vi "Internal Operation.vi"(7 "Archt Map":variant, 9 "Message":T2, 10 "ThreadData":T1={"AUTO_ERROR_HANDLE"={"ENABLE"=FALSE, "ANCHOR"="cleanup"}}, 11 "Numeric in":i32) -> (0 "error out":errorcluster, 2 "ThreadData (dup)":T1={"AUTO_ERROR_HANDLE"={"ENABLE"=FALSE, "ANCHOR"="cleanup"}}, 3 "Numeric out":i32)   [LabVIEW 2020, in "CSMScript-Engine(Lite).lvlib"]
uses:
  CSMScript-Engine(Lite).lvlib
  <userlib>/_NEVSTOP/Communicable State Machine(CSM)/addons/API-String-Arugments-Support/API String Arguments Support.lvlib
  <userlib>/_NEVSTOP/Communicable State Machine(CSM)/_Shared/CSM Shared.lvlib
  Typedef/Def-Thread Data.ctl
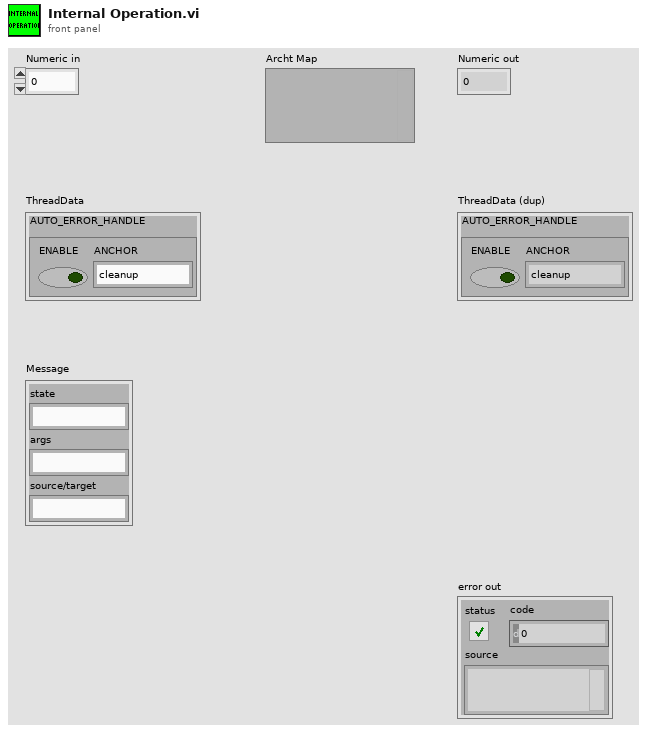
[diagram p1: front panel]
types:
  T1 = typedef "CSMScript-Engine(Lite).lvlib/Def-Thread Data.ctl" = cluster{"AUTO_ERROR_HANDLE":cluster{"ENABLE":bool, "ANCHOR":string}}
  T2 = cluster{"state":string, "args":string, "source/target":string}
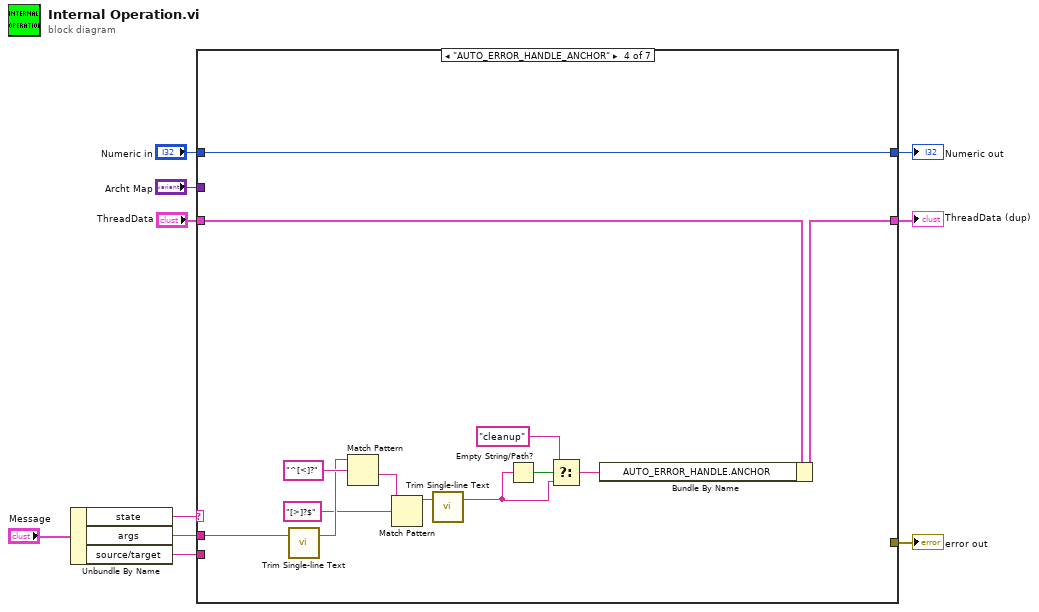
[diagram p0: block diagram]
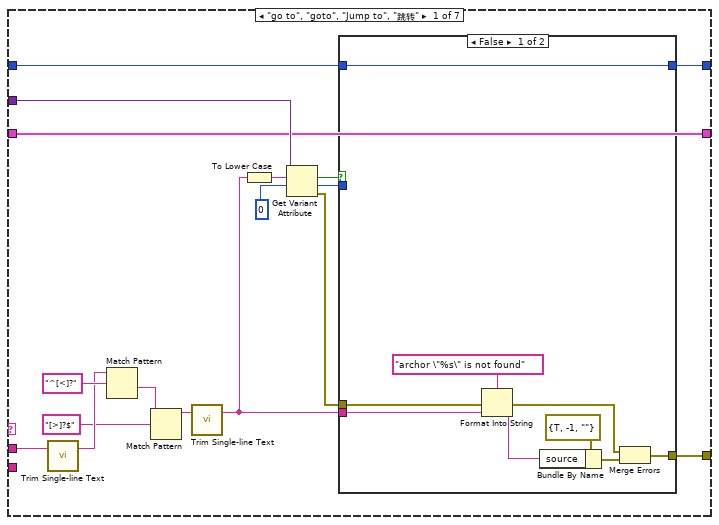
[diagram p2: hidden frame]
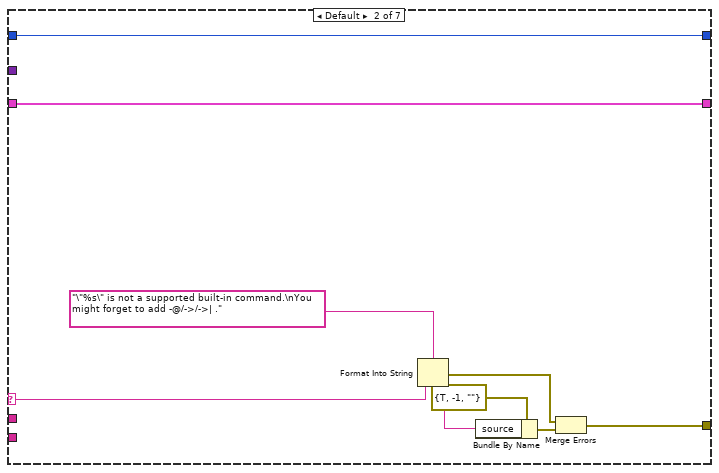
[diagram p4: hidden frame]
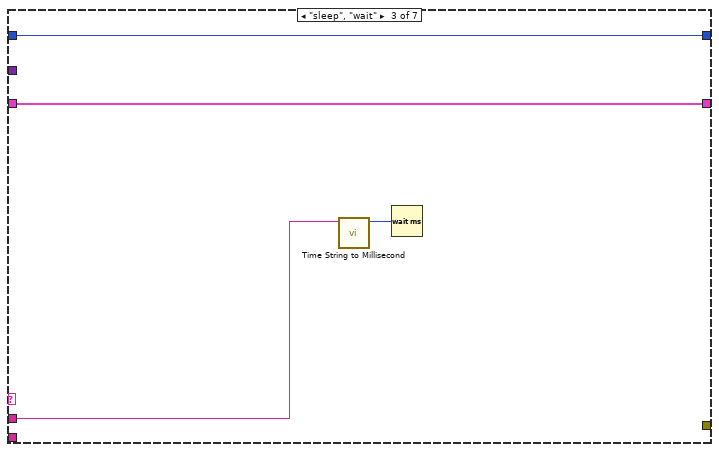
[diagram p5: hidden frame]
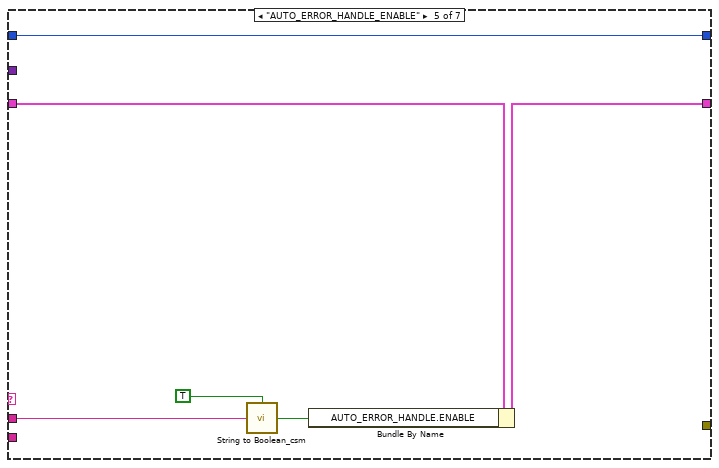
[diagram p6: hidden frame]
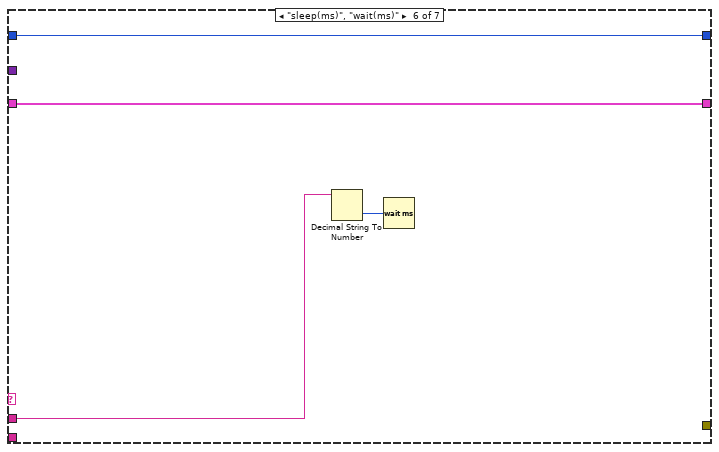
[diagram p7: hidden frame]
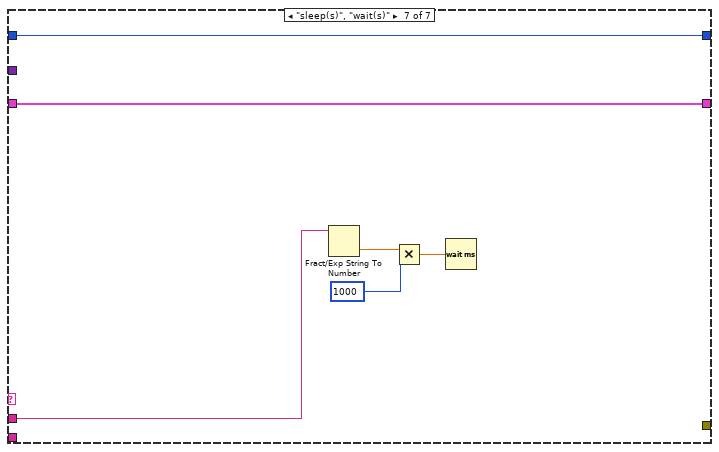
[diagram p8: hidden frame]
diagram:
  n1 = Unbundle By Name("Message") -> ("state"=w5:string, "args"=w4:string, "source/target"=w3:string)
  n2 = case shown="\"AUTO_ERROR_HANDLE_ANCHOR\"" w5 {
    selector: w5 -> [_ w39 _ _ _ _ _]
    tunnel: w4 -> [w17 _ w49 w52 w66 w72 w78]
    tunnel: [w24 w46 w50 w63 w69 w73 w79] -> w7
    tunnel: "Numeric in" -> [w23 w46 w50 w63 w69 w73 w79]
    tunnel: "Archt Map" -> [w27 _ _ _ _ _ _]
    tunnel: [w21 w40 _ _ _ _ _] -> w10
    tunnel: w3 -> [_ _ _ _ _ _ _]
    tunnel: "ThreadData" -> [w18 w38 w47 w62 w68 w70 w74]
    tunnel: [w18 w38 w47 w61 w67 w70 w74] -> w1
    frame "go to", "goto", "Jump to", "跳转" {
      n3 = call <userlib>:"Trim Single-line Text.vi"("single-line text"=w17) -> ("trimed text"=w15:string)  [unwired: 2 in]
      n4 = Match Pattern(string=w15, regular expression="^[<]?") -> (after substring=w13:string)  [unwired: 1 in, 3 out]
      n5 = Match Pattern(string=w13, regular expression="[>]?$") -> (before substring=w12:string)  [unwired: 1 in, 3 out]
      n6 = call <userlib>:"Trim Single-line Text.vi"("single-line text"=w12) -> ("trimed text"=w11:string)  [unwired: 2 in]
      n7 = To Lower Case(string=w11) -> (all lower case string=w19:string)
      n8 = Get Variant Attribute(Variant=w27, name=w19, default value (empty Variant)=0) -> (found=w22:bool, value=w25:i32, error out=w20:errorcluster)  [unwired: 1 in, 1 out]
      n9 = case shown="False" w22 {
        tunnel: w25 -> [_ w37]
        tunnel: [w28 w37] -> w24
        tunnel: w23 -> [w28 _]
        tunnel: w11 -> [w34 _]
        tunnel: [w30 _] -> w21
        tunnel: w20 -> [w31 _]
        frame False {
          n10 = Format Into String(format string="archor \"%s\" is not found" ("source"), error in=w31, w34) -> (resulting string=w33:string, error out=w29:errorcluster)  [unwired: 1 in]
          n11 = Bundle By Name(cluster=errorcluster {"status"=TRUE, "code"=-1, "source"=""} ("error in (no error)"), "source"=w33) -> (w32:errorcluster)
          n12 = Merge Errors(w29, w32) -> (w30:errorcluster)
        }
        frame True {
        }
      }
    }
    frame Default {
      n13 = Format Into String(format string="\"%s\" is not a supported built-in command.\nYou might forget to add -@/->/->| ." ("source"), w39) -> (resulting string=w43:string, error out=w41:errorcluster)  [unwired: 2 in]
      n14 = Bundle By Name(cluster=errorcluster {"status"=TRUE, "code"=-1, "source"=""} ("error in (no error)"), "source"=w43) -> (w42:errorcluster)
      n15 = Merge Errors(w41, w42) -> (w40:errorcluster)
    }
    frame "sleep", "wait" {
      n16 = call "Time String to Millisecond.vi"("Parameter"=w49) -> ("sum"=w48:i64)  [unwired: 8 in, 2 out]
      n17 = Wait (ms)(milliseconds to wait=w48) -> ()  [unwired: 1 out]
    }
    frame "AUTO_ERROR_HANDLE_ANCHOR" {
      n18 = call <userlib>:"Trim Single-line Text.vi"("single-line text"=w52) -> ("trimed text"=w56:string)  [unwired: 2 in]
      n19 = Match Pattern(string=w56, regular expression="^[<]?") -> (after substring=w54:string)  [unwired: 1 in, 3 out]
      n20 = Match Pattern(string=w54, regular expression="[>]?$") -> (before substring=w53:string)  [unwired: 1 in, 3 out]
      n21 = call <userlib>:"Trim Single-line Text.vi"("single-line text"=w53) -> ("trimed text"=w51:string)  [unwired: 2 in]
      n22 = Empty String/Path?(string/path=w51) -> (empty?=w60:bool)
      n23 = Select(t="cleanup", s=w60, f=w51) -> (s? t:f=w58:string)
      n24 = Bundle By Name(cluster=w62, "AUTO_ERROR_HANDLE.ANCHOR"=w58) -> (w61:T1)
    }
    frame "AUTO_ERROR_HANDLE_ENABLE" {
      n25 = call <userlib>:"String to Boolean_csm.vi"("Default (F)"=TRUE, "String"=w66) -> ("Boolean"=w65:bool)  [unwired: 2 in]
      n26 = Bundle By Name(cluster=w68, "AUTO_ERROR_HANDLE.ENABLE"=w65) -> (w67:T1)
    }
    frame "sleep(ms)", "wait(ms)" {
      n27 = Decimal String To Number(string=w72) -> (number=w71:i32)  [unwired: 2 in, 1 out]
      n28 = Wait (ms)(milliseconds to wait=w71) -> ()  [unwired: 1 out]
    }
    frame "sleep(s)", "wait(s)" {
      n29 = Fract/Exp String To Number(string=w78) -> (number=w77:dbl)  [unwired: 3 in, 1 out]
      n30 = Multiply(x=w77, y=1000) -> (x*y=w76:dbl)
      n31 = Wait (ms)(milliseconds to wait=w76) -> ()  [unwired: 1 out]
    }
  }
  "error out" <- w10
  "Numeric out" <- w7
  "ThreadData (dup)" <- w1
